vi "Create PVConnections.vi"(8 "Error In":errorcluster, 10 "PV-Infos":T1(array[cluster]), 11 "Object Name":string) -> (0 "error out":errorcluster, 3 "PVConnections":refnum<class "PVConnection.lvclass">[](array[class]))   [LabVIEW 2016, in "CS++ProcessVariables.lvlib"]
doc: "Create PVConnection objects."
uses:
  CS++ProcessVariables.lvlib
  PVConnection/PVConnection.lvclass
  C:/User/Brand/LVP/CSPP/Packages/CSPP_Core/Classes/CS++BaseClasses/Base/CS++Base.lvclass
  ProcessVariable/PV.lvclass
  ProcessVariable/PV.lvclass/PV.ctl
  CS++BaseClasses/Base/CS++Base.lvclass/CS++Base.ctl
  ProcessVariable/Write Type Descriptor.vi
  ProcessVariable/Write PV URL.vi
  ProcessVariable/Write Name.vi
  <vilib>/Utility/error.llb/Error Cluster From Error Code.vi
  CS++BaseClasses/Base/CS++Base.lvclass
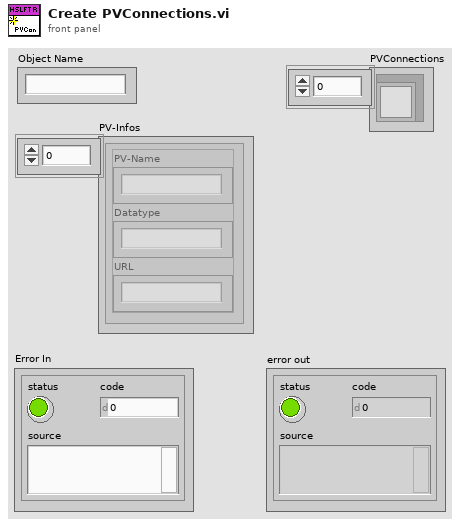
[diagram p1: front panel]
types:
  T1 = cluster{"PV-Name":string, "Datatype":string, "URL":string}[]
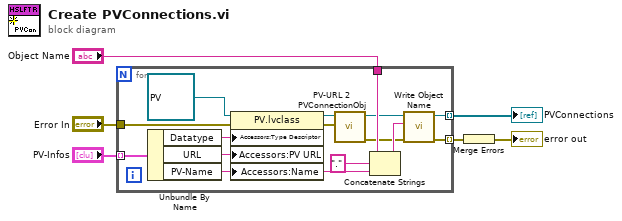
[diagram p0: block diagram]
diagram:
  n1 = for {
    tunnel: "PV-Infos" -> [w21] mode=indexing
    tunnel: "Object Name" -> [w14]
    tunnel: [w10] -> w6 mode=indexing
    tunnel: [w9] -> w4 mode=indexing
    tunnel: "Error In" -> [w7]
    n2 = Unbundle By Name(w21) -> ("Datatype"=w20:string, "URL"=w17:string, "PV-Name"=w15:string)
    n3 = property class="PV.lvclass"(reference=refnum<class "PV.lvclass"> refnum ("CS++ProcessVariables.lvlib:PV.lvclass"), error in=w7, "Accessors:Type Descriptor"=w20, "Accessors:PV URL"=w17, "Accessors:Name"=w15) -> (reference out=w19:refnum<class "PV.lvclass">, error out=w18:errorcluster)
    n4 = call "PV-URL 2 PVConnectionObj.vi"("Error In"=w18, "PV"=w19) -> ("Error Out"=w11:errorcluster, "PVConnection"=w13:refnum<class "PVConnection.lvclass">)  [unwired: 7 in, 1 out]
    n5 = Concatenate Strings(w14, "." ("string"), w15) -> (w12:string)
    n6 = call "Write Object Name.vi"("error in (no error)"=w11, "Object Name"=w12, "Base in"=w13) -> ("error out"=w9:errorcluster, "Base out"=w10:refnum<class "PVConnection.lvclass">)  [unwired: 7 in]
  }
  "PVConnections" <- w6
  n7 = Merge Errors(w4) -> (→"error out":errorcluster)
